vi "VI_FP controls to default values.vi"(8 "error in (no error)":errorcluster, 11 "VI in":refnum<vi>) -> (0 "error out":errorcluster, 3 "VI out":refnum<vi>)   [LabVIEW 2014]
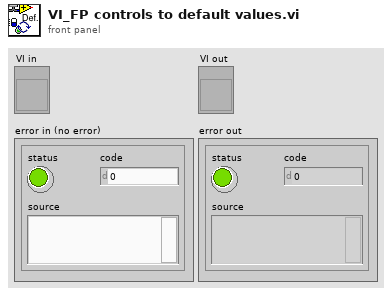
[diagram p1: front panel]
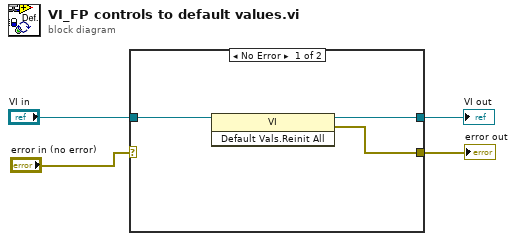
[diagram p0: block diagram]
diagram:
  n1 = case shown="No Error" "error in (no error)" {
    selector: "error in (no error)" -> [_ w8]
    tunnel: [w7 w9] -> w4
    tunnel: "VI in" -> [w6 w9]
    tunnel: [w5 w8] -> w1
    frame No Error {
      n2 = invoke class="VI" method="Default Vals.Reinit All"(reference=w6) -> (reference out=w7:refnum<vi>, error out=w5:errorcluster)  [unwired: 2 in, 1 out]
    }
    frame Error {
    }
  }
  "VI out" <- w4
  "error out" <- w1
